vi "dac_wavepara.vi"(8 "trigger_mode":enum16{"AUTO", "SOFT", "HARD"}(ring), 9 "frequency":dbl, 10 "cycles":u32, 11 "buf":dbl[](array[numeric])=[1.0]) -> (2 "wavepara":T1={"buf "=[1.0], "buflen"=0, "cycles"=0, "frequency"=0.0, "trigger_mode"=1})   [LabVIEW 2010, in "libdaqVI.lvlib"]
uses:
  libdaqVI.lvlib
panel:
  in  "wavepara":T1={"buf "=[1.0], "buflen"=0, "cycles"=0, "frequency"=0.0, "trigger_mode"=1}
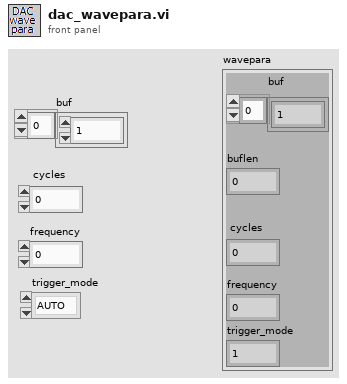
[diagram p1: front panel]
types:
  T1 = cluster{"buf ":dbl[], "buflen":u32, "cycles":u32, "frequency":dbl, "trigger_mode":u8}
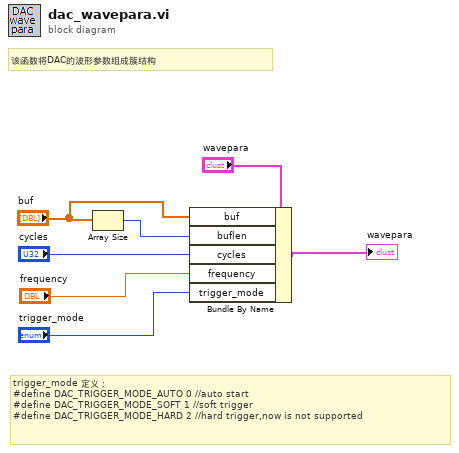
[diagram p0: block diagram]
diagram:
  # "该函数将DAC的波形参数组成簇结构"
  # "trigger_mode 定义：\n#define DAC_TRIGGER_MODE_AUTO 0 //auto start\n#define DAC_TRIGGER_MODE_SOFT 1 //soft trigger\n#define DAC_TRIGGER_MODE_HARD 2 //hard trigger,now is not supported"
  n1 = Array Size(array="buf") -> (size(s)=w6:i32)
  n2 = Bundle By Name(cluster="wavepara", "buf"="buf", "buflen"=w6, "cycles"="cycles", "frequency"="frequency", "trigger_mode"="trigger_mode") -> (→"wavepara":T1)
